vi "AO init.vi"(7 "N_moduls":i32, 10 "N_param":i32) -> (0 "error":errorcluster, 3 "AO":T1)   [LabVIEW 2019, in "Inputs.lvlib"]
uses:
  Inputs.lvlib
  Ctl/AO.ctl
  Ctl/Parameter State.ctl
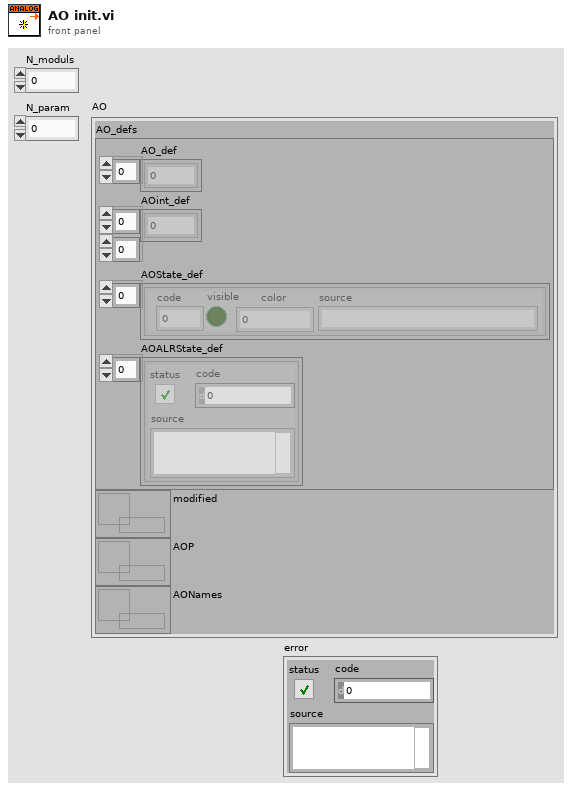
[diagram p1: front panel]
types:
  T1 = typedef "Inputs.lvlib/AO.ctl" = cluster{"AO_defs":cluster{"AO_def":dbl[], "AOint_def":u16[][], "AOState_def":T2[], "AOALRState_def":errorcluster[]}, "modified":refnum<data-value>, "AOP":refnum<data-value>, "AONames":refnum<data-value>}
  T2 = typedef "Inputs.lvlib/Parameter State.ctl" = cluster{"code":i32, "visible":bool, "color":u32, "source":string}
  T3 = cluster{"AO_def":dbl[], "AOint_def":u16[][], "AOState_def":T2[], "AOALRState_def":errorcluster[]}
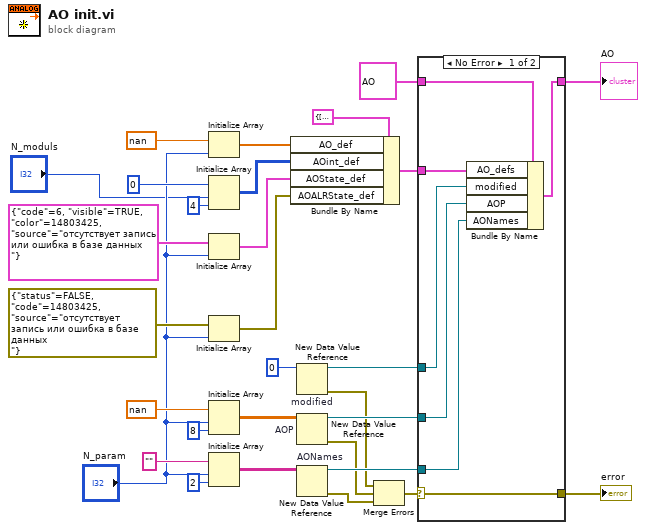
[diagram p0: block diagram]
diagram:
  n1 = Initialize Array(nan ("PV"), "N_param") -> (w28:dbl[])
  n2 = Initialize Array(u16 0 ("PV"), "N_moduls", 4 ("dimension size")) -> (w11:u16[][])
  n3 = Initialize Array(T2 {"code"=6, "visible"=TRUE, "color"=14803425, "source"="отсутствует запись или ошибка в базе данных                                                                                    "} ("STATE"), "N_param") -> (w12:T2[])
  n4 = Initialize Array(errorcluster {"status"=FALSE, "code"=14803425, "source"="отсутствует запись или ошибка в базе данных                                                                                    "} ("ALRSTATE"), "N_param") -> (w13:errorcluster[])
  n5 = Initialize Array(nan ("AOP"), "N_param", 8 ("dimension size")) -> (w8:dbl[][])
  n6 = Initialize Array("" ("AINames"), "N_param", 2 ("dimension size")) -> (w22:string[][])
  n7 = Bundle By Name(cluster=T3 {"AO_def"=[], "AOint_def"=[], "AOState_def"=[], "AOALRState_def"=[]} ("AO_defs"), "AO_def"=w28, "AOint_def"=w11, "AOState_def"=w12, "AOALRState_def"=w13) -> (w19:T3)
  n8 = New Data Value Reference "modified"(data value=u8 0 ("modified")) -> (data value reference=w2:refnum<data-value>, error out=w5:errorcluster)  [unwired: 1 in]
  n9 = New Data Value Reference "AOP"(data value=w8) -> (data value reference=w7:refnum<data-value>, error out=w4:errorcluster)  [unwired: 1 in]
  n10 = New Data Value Reference "AONames"(data value=w22) -> (data value reference=w21:refnum<data-value>, error out=w3:errorcluster)  [unwired: 1 in]
  n11 = Merge Errors(w5, w4, w3) -> (w6:errorcluster)
  n12 = case shown="No Error" w6 {
    selector: w6 -> [w34 w39]
    tunnel: w7 -> [w32 _]
    tunnel: w21 -> [w33 _]
    tunnel: [w34 w39] -> w20
    tunnel: w19 -> [w36 _]
    tunnel: T1 {"AO_defs"={"AO_def"=[], "AOint_def"=[], "AOState_def"=[], "AOALRState_def"=[]}, "modified"=refnum, "AOP"=refnum, "AONames"=refnum} ("AO") -> [w37 w38]
    tunnel: [w35 w38] -> w17
    tunnel: w2 -> [w31 _]
    frame No Error {
      n13 = Bundle By Name(cluster=w37, "AO_defs"=w36, "modified"=w31, "AOP"=w32, "AONames"=w33) -> (w35:T1)
    }
    frame Error {
    }
  }
  "error" <- w20
  "AO" <- w17
